vi "Multimeter_ReadData.vi"(8 "error in (no error)":errorcluster, 11 "MultimeterControl in":refnum<class "MultimeterControl.lvclass">) -> (0 "error out":errorcluster, 2 "Voltage in V":dbl, 3 "MultimeterControl out":refnum<class "MultimeterControl.lvclass">)   [LabVIEW 2019, in "MultimeterControl.lvclass"]
uses:
  MultimeterControl.lvclass
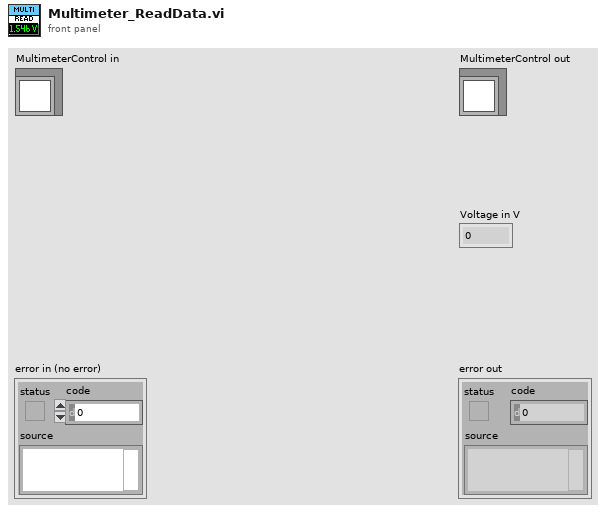
[diagram p1: front panel]
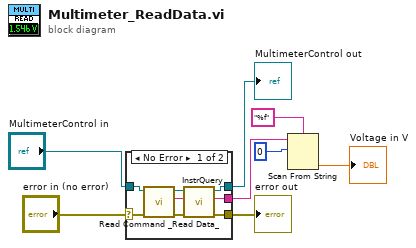
[diagram p0: block diagram]
diagram:
  n1 = case shown="No Error" "error in (no error)" {
    selector: "error in (no error)" -> [w9 w18]
    tunnel: [w15 w18] -> w7
    tunnel: [w16 w17] -> w5
    tunnel: "MultimeterControl in" -> [w10 w17]
    tunnel: [w14 _] -> w2
    frame No Error {
      n2 = call-dynamic "Read Command _Read Data_.vi"("error in (no error)"=w9, "MultimeterControl in"=w10) -> ("error out"=w11:errorcluster, "Command \"Read Data\""=w12:string, "MultimeterControl out"=w13:refnum<class "MultimeterControl.lvclass">)  [unwired: 7 in]
      n3 = call-dynamic "InstrQuery.vi"("error in (no error)"=w11, "Command string"=w12, "InstControl in"=w13) -> ("error out"=w15:errorcluster, "Instrument response"=w14:string, "InstControl out"=w16:refnum<class "MultimeterControl.lvclass">)  [unwired: 6 in]
    }
    frame Error {
    }
  }
  "error out" <- w7
  "MultimeterControl out" <- w5
  n4 = Scan From String(format string="%f", input string=w2, initial scan location=0) -> (output 1=→"Voltage in V":dbl)  [unwired: 2 in, 3 out]
